vi "Audit Trail Insert data.vi"(8 "error in (no error)":errorcluster, 9 "Activity":string, 10 "User":string, 11 "connection reference":T1) -> (0 "error out":errorcluster)   [LabVIEW 2018]
uses:
  <vilib>/addons/database/Connection.llb/Conn ObjectReference.ctl
  <vilib>/addons/database/NI_Database_API.lvlib
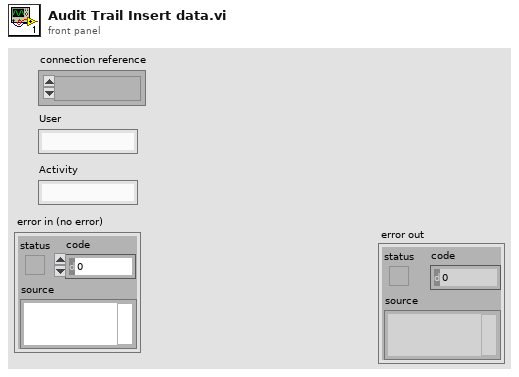
[diagram p1: front panel]
types:
  T1 = typedef "NI_Database_API.lvlib/Conn ObjectReference.ctl" = refnum<k1>
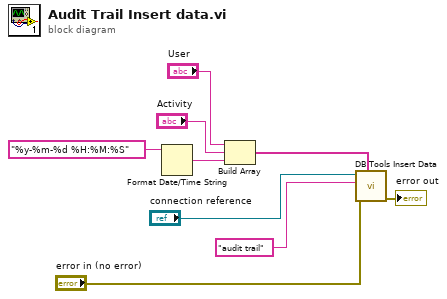
[diagram p0: block diagram]
diagram:
  n1 = Format Date/Time String(time format string (%c)="%y-%m-%d %H:%M:%S") -> (date/time string=w5:string)  [unwired: 2 in]
  n2 = Build Array("User", "Activity", w5) -> (w4:string[])
  n3 = call <vilib>:"DB Tools Insert Data.vi"("data"=w4, "error in (no error)"="error in (no error)", "table"="audit trail", "connection reference"="connection reference") -> ("error out"=→"error out":errorcluster)  [unwired: 6 in, 1 out]
